vi "TriggerCheck.vi"(7 "SamplesOverThreshold":u8, 10 "TriggerLevel":i16, 11 "Acceleration":i16) -> (3 "Trigger?":bool)   [LabVIEW 2019]
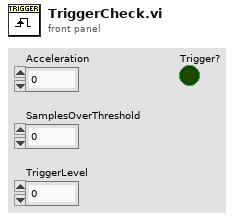
[diagram p1: front panel]
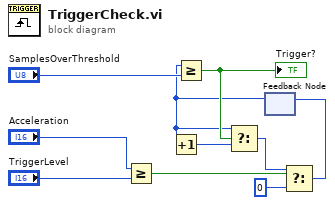
[diagram p0: block diagram]
diagram:
  n1 = Greater Or Equal?(x="Acceleration", y="TriggerLevel") -> (x >= y?=w7:bool)
  n2 = feedback #1() -> (w1:u8)  [unwired: 1 in]
  n3 = Increment(x=w1) -> (x+1=w4:u8)
  n4 = Greater Or Equal?(x=w1, y="SamplesOverThreshold") -> (x >= y?=w2:bool)
  "Trigger?" <- w2
  n5 = Select(t=w1, s=w2, f=w4) -> (s? t:f=w3:u8)
  n6 = Select(t=w3, s=w7, f=u8 0) -> (s? t:f=w9:u8)
  n7 = feedback-in #1(w9) -> ()
